vi "Write to DB Post-Assembly.vi"(8 "error in (no error)":errorcluster, 10 "Stack names":T1, 11 "Database Entry in":refnum<class "Database Entry.lvclass">) -> (0 "error out":errorcluster, 3 "Database Entry out":refnum<class "Database Entry.lvclass">)   [LabVIEW 2021, in "Database Entry.lvclass"]
uses:
  Database Entry.lvclass
  Database Entry.lvclass/Database Entry.ctl
  <vilib>/Utility/file.llb/Read Delimited Spreadsheet (string).vi
  <vilib>/Utility/file.llb/Write Delimited Spreadsheet (string).vi
  Components/Stack/Stack.lvclass
panel:
  out "error out py":errorcluster
  out "String Out":string="Upload Success"
  out "Data cluster":T2={"module or proto"="proto", "stack name"="some", "timeend"="1:23:45.244", "Comments"=""}
  in  "error in (no error) py":errorcluster
  # "Debug instructions\n#### The order of values in db_data_cols must match the order of values in Data cluster in Stack.lvclass: Get stack data.vi \n#### The variable names below correspond to postgres col name. LV does not neet to match the col numes but just the values. \n#### Right-click on the Data cluster on the front panel and click on 'reorder controls' to verify the order is correct in the code. \n#### The physical position of the fields is different from the actual position.\n\nIn Main VIs/python_db/postgres_tools.py, see functions 'assembly_data' and 'assembly_data_as_list'."
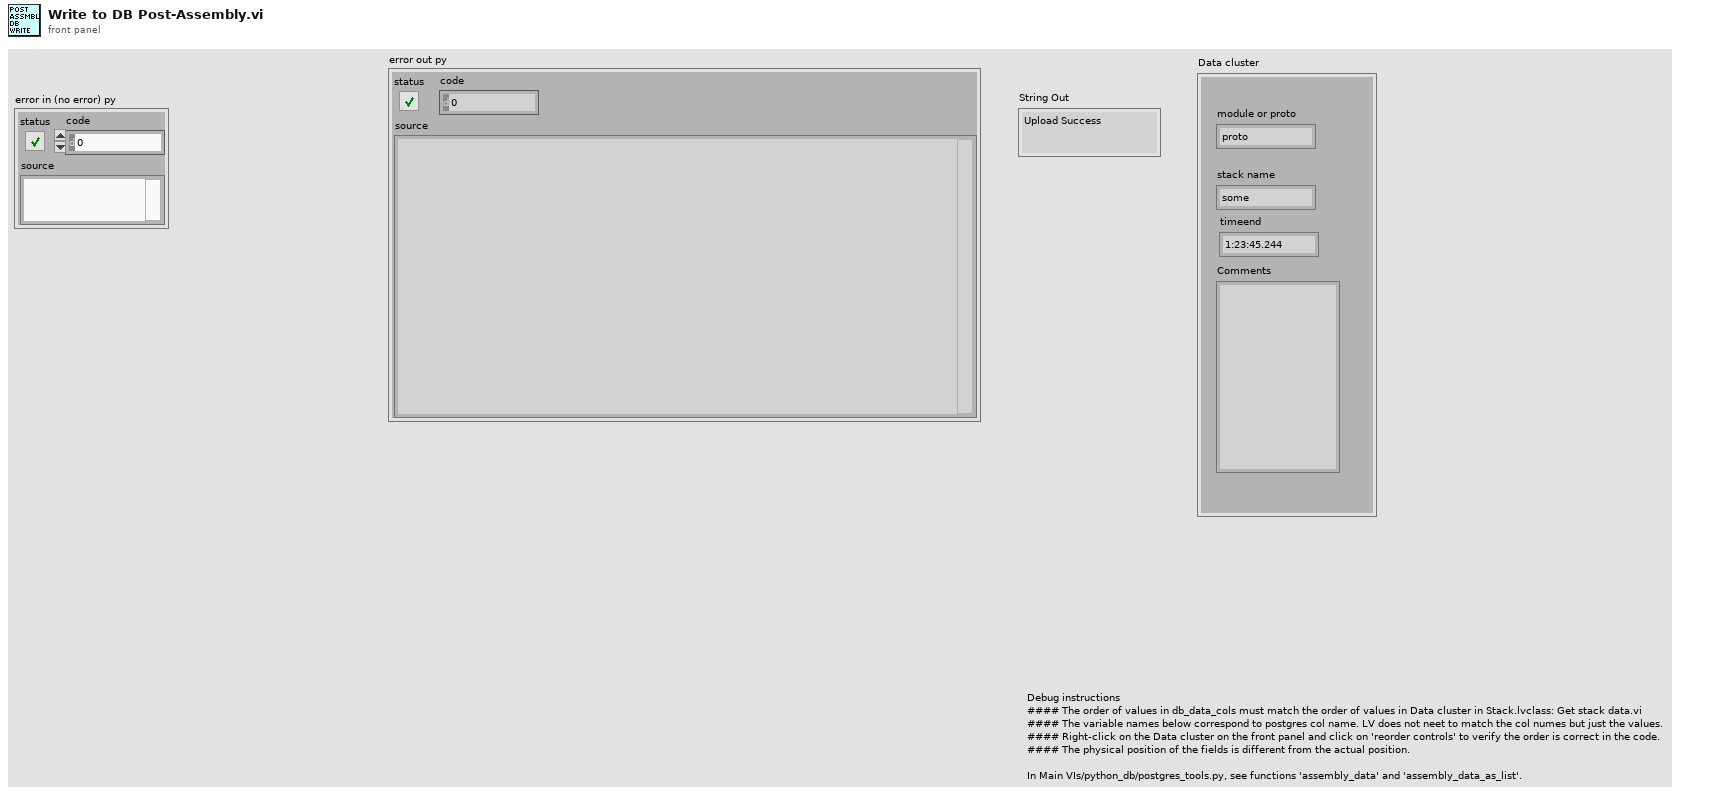
[diagram p1: front panel]
types:
  T1 = cluster{"(1) Tray 1 Pos 1":string, "(2) Tray 1 Pos 2":string, "(3) Tray 2 Pos 1":string, "(4) Tray 2 Pos 2":string}
  T2 = cluster{"module or proto":string, "stack name":string, "timeend":string, "Comments":string}
  T3 = typedef "File Paths.ctl" = cluster{"Glue Pattern Folder":path, "Carrier Tray Folder":path, "Pick Up Tool Fixture Folder":path, "Components Folder":path, "Bellows Tool Offset.txt":path, "Pick Up Tool Offset.txt":path, "Dispense Tip Offset.txt":path, "Log Files":path, "Gantry Assembly Map.txt":path, "Syringe and offset map.txt":path, "Controllers Folder":path, "Local dbase config":path}
  T4 = cluster{"(1) Tray 1 Pos 1":cluster{"Stack name":string, "Post-assembly comments":string}, "(2) Tray 1 Pos 2":cluster{"Stack name":string, "Post-assembly comments":string}, "(3) Tray 2 Pos 1":cluster{"Stack name":string, "Post-assembly comments":string}, "(4) Tray 2 Pos 2":cluster{"Stack name":string, "Post-assembly comments":string}}
  T5 = cluster{"Stack name":string, "Post-assembly comments":string}[]
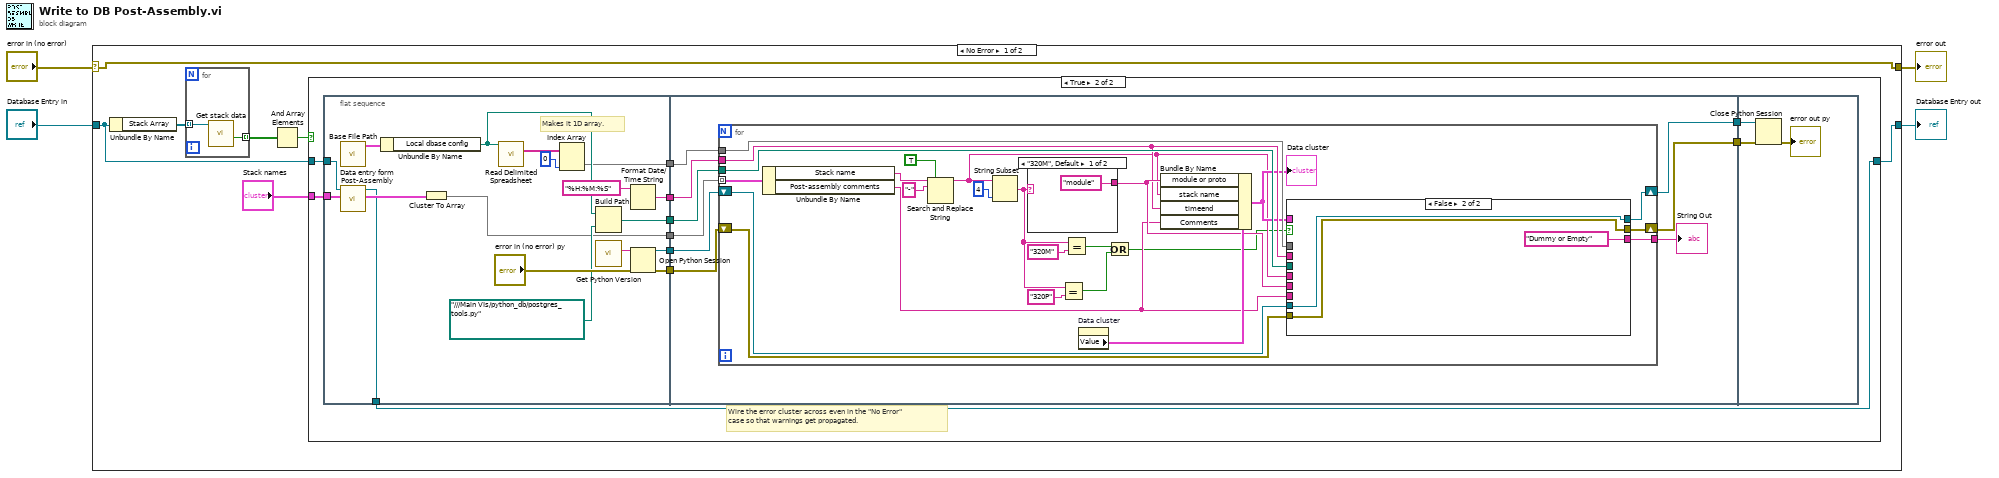
[diagram p0: block diagram]
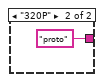
[diagram p3: hidden frame]
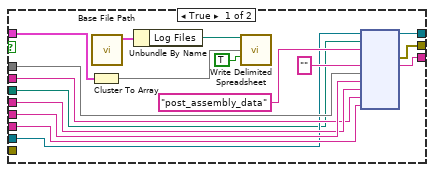
[diagram p4: hidden frame]
diagram:
  n1 = case shown="No Error" "error in (no error)" {
    selector: "error in (no error)" -> [w9 w102]
    tunnel: "Database Entry in" -> [w8 w103]
    tunnel: [w10 w103] -> w2
    tunnel: [w9 w102] -> w1
    frame No Error {
      n2 = Unbundle By Name(w8) -> ("Stack Array"=w7:refnum<class "Stack.lvclass">[])
      n3 = for {
        tunnel: w7 -> [w101] mode=indexing
        tunnel: [w100] -> w6 mode=indexing
        n4 = call "Get stack data.vi"("Stack in"=w101) -> ("Is real run"=w100:bool)  [unwired: 7 in, 3 out]
      }
      n5 = And Array Elements(Boolean array=w6) -> (logical AND=w5:bool)
      n6 = case shown="True" w5 {
        tunnel: "Stack names" -> [_ w15]
        tunnel: w8 -> [w12 w14]
        tunnel: [w12 w13] -> w10
        frame False {
        }
        frame True {
          # "Wire the error cluster across even in the \"No Error\"\ncase so that warnings get propagated."
          n7 = flat-sequence {
            tunnel: [w40] -> w23
            tunnel: [w41] -> w22
            tunnel: [w37] -> w21
            tunnel: [w33] -> w20
            tunnel: [w30] -> w19
            tunnel: [w28] -> w18
            tunnel: w15 -> [w26]
            tunnel: w14 -> [w25]
            tunnel: [w24] -> w13
            tunnel: [w49] -> w17
            tunnel: [w48] -> w16
            tunnel: w23 -> [w50]
            tunnel: w22 -> [w47]
            tunnel: w21 -> [w46]
            tunnel: w20 -> [w45]
            tunnel: w19 -> [w43]
            tunnel: w18 -> [w42]
            tunnel: w17 -> [w98]
            tunnel: w16 -> [w99]
            frame #0 {
              # "Makes it 1D array."
              n8 = call "Base File Path.vi"() -> ("Paths Out"=w38:T3)  [unwired: 11 in]
              n9 = call "Data entry form Post-Assembly.vi"("Stack names"=w26, "Database Entry in"=w25) -> ("Post-Assembly Comments Out"=w27:T4, "Database Entry out"=w24:refnum<class "Database Entry.lvclass">)  [unwired: 7 in, 1 out]
              n10 = Unbundle By Name(w38) -> ("Local dbase config"=w36:path)
              n11 = Cluster To Array(cluster=w27) -> (array=w30:T5)
              n12 = call-poly <vilib>:"Read Delimited Spreadsheet.vi"("file path (dialog if empty)"=w36) -> ("all rows"=w35:string[][])  [unwired: 9 in, 5 out]
              n13 = Index Array(array=w35, index (col)=0 ("disabled index (col)")) -> (element=w33:string[])  [unwired: 1 in]
              n14 = Build Path(base path=w36, name or relative path=path "../../../Main VIs/python_db/postgres_tools.py" ("module path")) -> (appended path=w37:path)
              n15 = call "Get Python Version.vi"() -> ("Python Version"=w31:string)  [unwired: 10 in, 1 out]
              n16 = Format Date/Time String(time format string (%c)="%H:%M:%S") -> (date/time string=w28:string)  [unwired: 2 in]
              n17 = Open Python Session(python version=w31, 3:"error in (no error) py") -> (session out=w41:refnum<k35>, error out=w40:errorcluster)  [unwired: 1 in]
            }
            frame #1 {
              n18 = for {
                tunnel: w46 -> [w69]
                shift-right: [w74] -> w49
                shift-left: w50 -> [w68]
                shift-right: [w73] -> w48
                shift-left: w47 -> [w70]
                tunnel: [w72] -> w44
                tunnel: w45 -> [w71]
                tunnel: w43 -> [w67] mode=indexing
                tunnel: w42 -> [w63]
                n19 = Unbundle By Name(w67) -> ("Stack name"=w59:string, "Post-assembly comments"=w62:string)
                n20 = Search and Replace String(replace all?=TRUE ("replace all? (F)"), input string=w59, search string="-") -> (result string=w60:string)  [unwired: 5 in, 3 out]
                n21 = String Subset(string=w60, length (rest)=4 ("length (rest)")) -> (substring=w52:string)  [unwired: 1 in]
                n22 = case shown="\"320M\", Default" w52 {
                  tunnel: ["module" "proto"] -> w64
                  frame "320M", Default {
                  }
                  frame "320P" {
                  }
                }
                n23 = Equal?(x=w52, y="320P") -> (x = y?=w53:bool)
                n24 = Equal?(x=w52, y="320M") -> (x = y?=w54:bool)
                n25 = property on="Data cluster" class="Clust (strict)"() -> ("Value"=w66:T2)  [unwired: 2 in, 2 out]
                n26 = Or(x=w54, y=w53) -> (x .or. y?=w51:bool)
                n27 = Bundle By Name(cluster=w66, "module or proto"=w64, "stack name"=w60, "timeend"=w63, "Comments"=w62) -> (w61:T2)
                "Data cluster" <- w61
                n28 = case shown="False" w51 {
                  tunnel: [w93 w96] -> w74
                  tunnel: [w92 w94] -> w73
                  tunnel: [w91 "Dummy or Empty"] -> w72
                  tunnel: w71 -> [w89 _]
                  tunnel: w70 -> [w78 w94]
                  tunnel: w69 -> [w77 _]
                  tunnel: w68 -> [_ w96]
                  tunnel: w64 -> [w84 _]
                  tunnel: w60 -> [w83 _]
                  tunnel: w63 -> [w82 _]
                  tunnel: w62 -> [w81 _]
                  tunnel: w61 -> [w80 _]
                  frame True {
                    n29 = Cluster To Array(cluster=w80) -> (array=w79:string[])
                    n30 = call "Base File Path.vi"() -> ("Paths Out"=w87:T3)  [unwired: 11 in]
                    n31 = Unbundle By Name(w87) -> ("Log Files"=w86:path)
                    n32 = call-poly <vilib>:"Write Delimited Spreadsheet.vi"("file path (dialog if empty)"=w86, "1D data"=w79, "append to file? (new file:F)"=TRUE) -> ()  [unwired: 11 in, 2 out]
                    n33 = node(w78, w77, "post_assembly_data" ("function name"), "", w89, w84, w83, w82, w81) -> (w92:refnum<k35>, w93:errorcluster, w91:string)  [unwired: 6 in, 2 out]
                  }
                  frame False {
                  }
                }
              }
              "String Out" <- w44
            }
            frame #2 {
              n34 = Close Python Session(session in=w99, error in=w98) -> (11:→"error out py":errorcluster)
            }
          }
        }
      }
    }
    frame Error {
    }
  }
  "Database Entry out" <- w2
  "error out" <- w1
